vi "CleanUp.vi"(8 "Error In":errorcluster, 11 "object in":refnum<class "GameEl.lvclass">) -> (0 "Error Out":errorcluster, 3 "object out":refnum<class "GameEl.lvclass">)   [LabVIEW 2021, in "GameEl.lvclass"]
uses:
  GameEl.lvclass
  GameEl.lvclass/GameEl.ctl
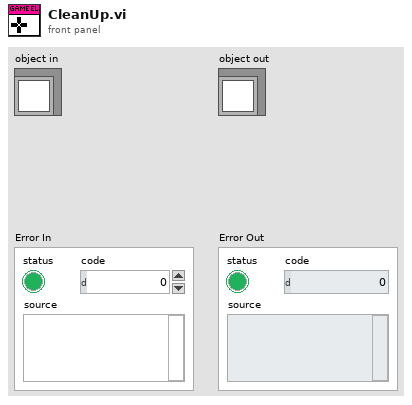
[diagram p1: front panel]
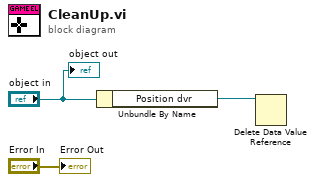
[diagram p0: block diagram]
diagram:
  n1 = Unbundle By Name("object in") -> ("Position dvr"=w2:refnum<data-value>)
  n2 = Delete Data Value Reference(data value reference=w2) -> ()  [unwired: 1 in, 2 out]
  "Error Out" <- "Error In"
  "object out" <- "object in"
